vi "ROI构造器.vi"() -> ()   [LabVIEW 2018]
panel:
  out "error out":errorcluster
  out "ROI Descriptor Out":T1 {"Contours"."Type" items=["No Selection", "Point", "Line", "Rectangle", "Oval", "Polygon", "Freehand Region", "Annulus", "Unused2", "Unused3", "Broken Line", "Freehand Line", "Rotated Rectangle"]}
  in  "结束":bool
  in  "清楚ROI":bool
  in  "创建ROI":bool
  in  "显示图像":bool
  in  "路径":path
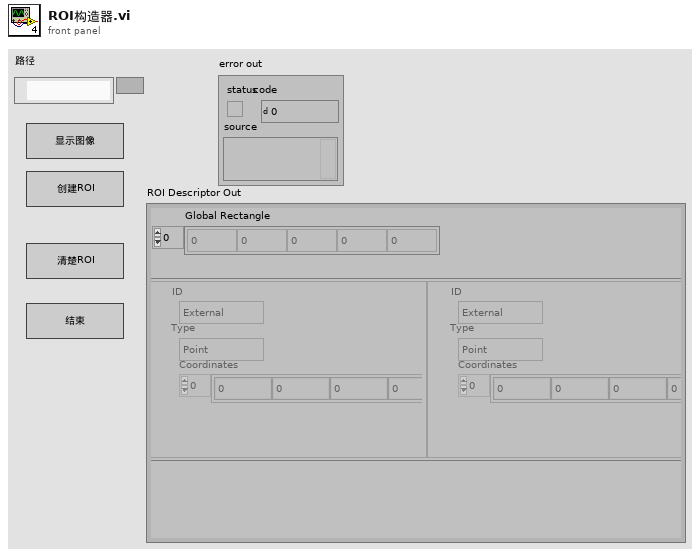
[diagram p1: front panel]
types:
  T1 = typedef "ROI Descriptor" = cluster{"Global Rectangle":i32[], "Contours":cluster{"ID":enum32{"External", "Internal"}, "Type":u32, "Coordinates":i32[]}[]}
  T2 = typedef "Image Type" = u32
  T3 = typedef "IMAQ Image.ctl" = refnum<image>
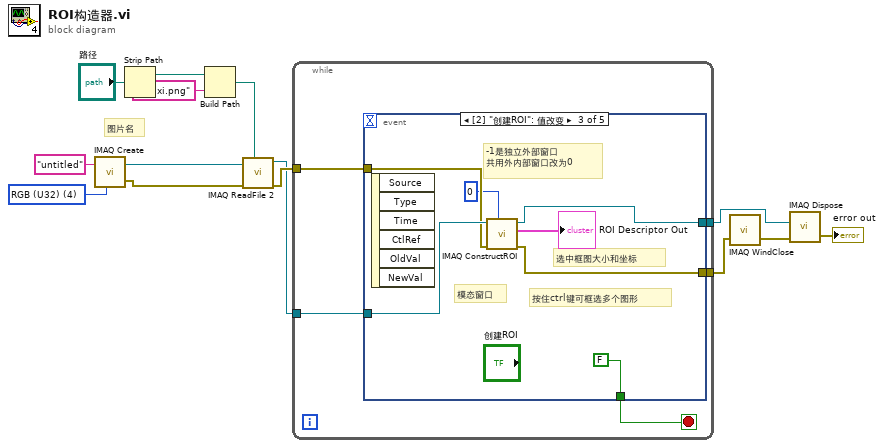
[diagram p0: block diagram]
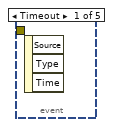
[diagram p2: hidden frame]
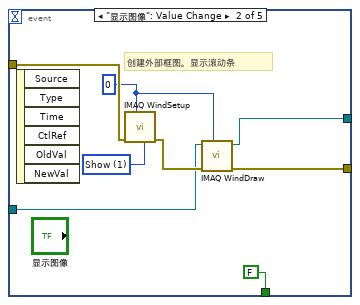
[diagram p3: hidden frame]
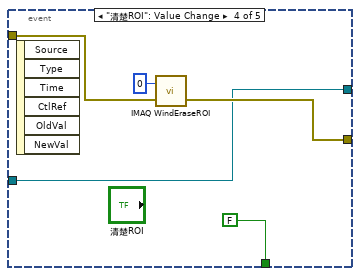
[diagram p4: hidden frame]
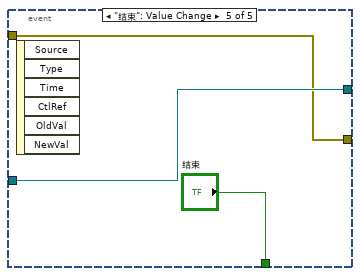
[diagram p5: hidden frame]
diagram:
  w8 = T2 4 items=["Grayscale (U8)", "Grayscale (I16)", "Grayscale (SGL)", "Complex (CSG)", "RGB (U32)", "HSL (U32)", "RGB (U64)", "Grayscale (U16)"] ("Image Type")
  # "图片名"
  n1 = call "IMAQ Create"("Image Name"="untitled", "Image Type"=w8) -> ("New Image"=w10:T3, "error out"=w9:errorcluster)  [unwired: 3 in]
  n2 = Strip Path(path="路径") -> (stripped path=w14:path)  [unwired: 1 out]
  n3 = Build Path(base path=w14, name or relative path="lainxi.png" ("名称或相对路径")) -> (appended path=w7:path)
  n4 = call "IMAQ ReadFile 2"("File Path"=w7, "error in (no error)"=w9, "Image"=w10) -> ("error out"=w6:errorcluster, "Image Out"=w2:T3)  [unwired: 4 in, 3 out]
  n5 = while {
    tunnel: w6 -> [w19]
    tunnel: [w18] -> w4
    tunnel: [w17] -> w5
    tunnel: w2 -> [w15]
    stop <- w16 stop-if-true
    n6 = event shown="[2] \"创建ROI\": 值改变" {
      selector: _ -> [_ _ _ _ _]
      dyn-events: _ -> [_ _ _ _ _]
      timeout: _ -> [_ _ _ _ _]
      tunnel: w19 -> [_ w27 w32 w39 w40]
      tunnel: [_ w23 w31 w37 w41] -> w18
      tunnel: [_ w22 w30 w38 w40] -> w17
      tunnel: [_ FALSE FALSE FALSE "结束"] -> w16
      tunnel: w15 -> [_ w20 w33 w37 w41]
      event Timeout {
        n7 = event-data() -> ()  [unwired: 1 in, 3 out]
      }
      event "显示图像": Value Change {
        w25 = 1 items=["Hide", "Show", "No change"] ("Scrollbars (No change)")
        w24 = 0 ("Window Number (0...15)")
        # "创建外部框图。显示滚动条"
        n8 = event-data() -> ()  [unwired: 1 in, 6 out]
        n9 = call "IMAQ WindSetup"("Scrollbars (No change)"=w25, "Window Number (0...15)"=w24, "error in (no error)"=w27) -> ("error out"=w26:errorcluster)  [unwired: 8 in]
        n10 = call "IMAQ WindDraw"("Window Number (0...15)"=w24, "error in (no error)"=w26, "Image"=w20) -> ("error out"=w22:errorcluster, "Image Out (duplicate)"=w23:T3)  [unwired: 7 in]
      }
      event "创建ROI": Value Change {
        # "按住ctrl键可框选多个图形"
        # "选中框图大小和坐标"
        # "模态窗口"
        # "-1是独立外部窗口\n共用外内部窗口改为0"
        n11 = event-data() -> ()  [unwired: 1 in, 6 out]
        n12 = call "IMAQ ConstructROI"("Window Number (-1...15)"=0, "error in (no error)"=w32, "Image"=w33) -> ("error out"=w30:errorcluster, "ROI Descriptor Out"=→"ROI Descriptor Out":T1, "Image Out (duplicate)"=w31:T3)  [unwired: 5 in, 1 out]
      }
      event "清楚ROI": Value Change {
        n13 = event-data() -> ()  [unwired: 1 in, 6 out]
        n14 = call "IMAQ WindEraseROI"("Window Number"=0, "error in (no error)"=w39) -> ("error out"=w38:errorcluster)  [unwired: 4 in]
      }
      event "结束": Value Change {
        n15 = event-data() -> ()  [unwired: 1 in, 6 out]
      }
    }
  }
  n16 = call "IMAQ WindClose"("error in (no error)"=w5) -> ("error out"=w3:errorcluster)  [unwired: 5 in]
  n17 = call "IMAQ Dispose"("Image"=w4, "error in (no error)"=w3) -> ("error out"=→"error out":errorcluster)  [unwired: 4 in]
